vi "Build Sparse Array.vi"(4 "Side":T1=enum."right") -> ()   [LabVIEW 2013]
uses:
  ROS/Code/SubVIs/BaxterSide.ctl
  Baxter Examples/Arm Globals.vi
  <vilib>/Utility/config.llb/Read Key (Double).vi
  Fwd Kenimatics - array.vi
  <vilib>/Utility/config.llb/NI_LVConfig.lvlib
panel:
  out "output variable":dbl
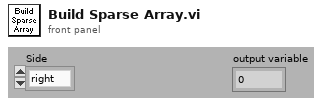
[diagram p1: front panel]
types:
  T1 = typedef "BaxterSide.ctl" = enum16{"left", "right"}
  T2 = cluster{"J[0]":dbl, "J[1]":dbl, "J[2]":dbl, "J[3]":dbl, "J[4]":dbl, "J[5]":dbl, "J[6]":dbl}
  T3 = cluster{"Label":string, "Joints":dbl[], "Far Left":cluster{"Absolute":dbl[], "Robot":dbl[]}, "Far Right":cluster{"Absolute":dbl[], "Robot":dbl[]}, "Near Left":cluster{"Absolute":dbl[], "Robot":dbl[]}, "Near Right":cluster{"Absolute":dbl[], "Robot":dbl[]}}[]
  T4 = typedef "NI_Matrix.lvlib/RealMatrix.ctl" = dbl[][]
  T5 = cluster{"Label":string, "Joints":dbl[], "T":T4}[]
  T6 = typedef "NI_LVConfig.lvlib/Config Data RefNum.ctl" = refnum<k1>
  T7 = cluster{"J[0]":dbl, "J[1]":dbl, "J[2]":dbl, "J[3]":dbl, "J[4]":dbl, "J[5]":dbl, "J[6]":dbl}[]
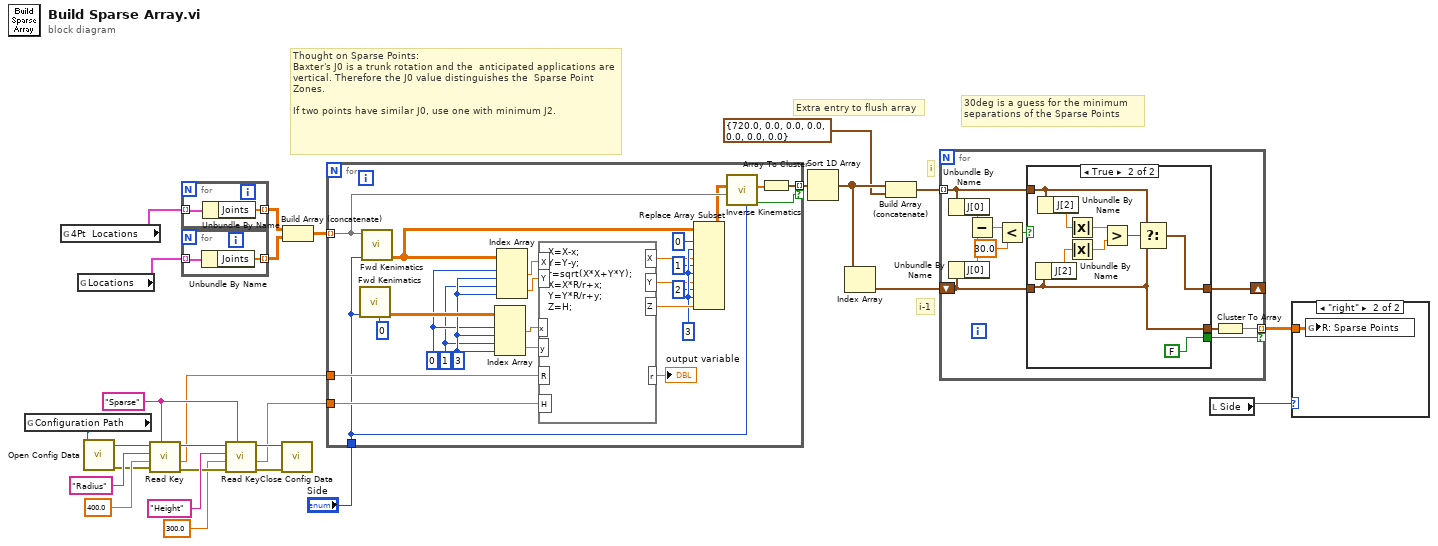
[diagram p0: block diagram]
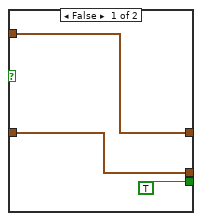
[diagram p3: hidden frame]
diagram:
  w23 = "Sparse"
  # "30deg is a guess for the minimum\nseparations of the Sparse Points"
  # "Extra entry to flush array"
  # "i-1"
  # "i"
  # "Thought on Sparse Points:\nBaxter's J0 is a trunk rotation and the  anticipated applications are vertical. Therefore the J0 value distinguishes the  Sparse Point Zones.\n\nIf two points have similar J0, use one with minimum J2."
  n1 = global read "Arm Globals.vi" "Configuration Path"() -> (w27:path)
  n2 = global read "Arm Globals.vi" "4Pt  Locations"() -> (w13:T3)
  n3 = global read "Arm Globals.vi" "Locations"() -> (w12:T5)
  n4 = call <vilib>:"Open Config Data.vi"("configuration file path"=w27) -> ("error out"=w20:errorcluster, "refnum"=w26:T6)  [unwired: 8 in, 1 out]
  n5 = call-poly <vilib>:"Read Key.vi"("section"=w23, "error in (no error)"=w20, "default value"=400.0, "key"="Radius", "refnum"=w26) -> ("error out"=w19:errorcluster, "value"=w15:dbl, "refnum out"=w24:T6)  [unwired: 3 in, 1 out]
  n6 = for {
    tunnel: w13 -> [w29] mode=indexing
    tunnel: [w28] -> w11 mode=indexing
    n7 = Unbundle By Name(w29) -> ("Joints"=w28:dbl[])
  }
  n8 = for {
    tunnel: w12 -> [w31] mode=indexing
    tunnel: [w30] -> w10 mode=indexing
    n9 = Unbundle By Name(w31) -> ("Joints"=w30:dbl[])
  }
  n10 = call-poly <vilib>:"Read Key.vi"("section"=w23, "error in (no error)"=w19, "default value"=300.0, "key"="Height", "refnum"=w24) -> ("error out"=w16:errorcluster, "value"=w14:dbl, "refnum out"=w17:T6)  [unwired: 3 in, 1 out]
  n11 = call <vilib>:"Close Config Data.vi"("error in (no error)"=w16, "refnum"=w17) -> ()  [unwired: 8 in, 2 out]
  n12 = Build Array (concatenate)(w11, w10) -> (w9:dbl[][])
  n13 = for {
    tunnel: w15 -> [w54]
    tunnel: w14 -> [w51]
    tunnel: w9 -> [w45] mode=indexing
    tunnel: "Side" -> [w33]
    tunnel: [w41] -> w8 mode=indexing if=w40
    w35 = 1 ("disabled index (row)")
    w36 = 0 ("disabled index (row)")
    w37 = 3 ("disabled index (col)")
    w48 = 3 ("disabled index (col)")
    n14 = call-poly "Fwd Kenimatics.vi"("To"=0, "Side"=w33) -> ("Matrix"=w38:T4)  [unwired: 8 in, 1 out]
    n15 = call-poly "Fwd Kenimatics.vi"("Side"=w33, "Joints"=w45) -> ("Matrix"=w34:T4)  [unwired: 8 in, 1 out]
    n16 = Index Array(array=w38, index (row) #1=w36, index (col) #1=w37, index (row) #2=w35, index (col) #2=w37) -> (element #1=w52:dbl, element #2=w53:dbl)
    n17 = Index Array(array=w34, index (row) #1=w36, index (col) #1=w37, index (row) #2=w35, index (col) #2=w37) -> (element #1=w56:dbl, element #2=w55:dbl)
    n18 = formula code="X=X-x;\nY=Y-y;\nr=sqrt(X*X+Y*Y);\nX=X*R/r+x;\nY=Y*R/r+y;\nZ=H;"("R"=w54, "X"=w56, "Y"=w55, "x"=w52, "y"=w53, "H"=w51) -> ("r"=→"output variable":dbl, "X"=w44:dbl, "Y"=w43:dbl, "Z"=w50:dbl)
    n19 = Replace Array Subset(array=w34, new element #1=w44, index (row) #1=0 ("disabled index (row)"), index (col) #1=w48, new element #2=w43, index (row) #2=1 ("disabled index (row)"), index (col) #2=w48, new element #3=w50, index (row) #3=2 ("disabled index (row)"), index (col) #3=w48) -> (w32:T4)
    n20 = call "Inverse Kinematics.vi"("Side"=w33, "Start"=w45, "Goal-matrix"=w32) -> ("Found"=w40:bool, "J"=w42:dbl[])  [unwired: 5 in, 2 out]
    n21 = Array To Cluster(array=w42) -> (cluster=w41:T2)
  }
  n22 = Sort 1D Array(array=w8) -> (sorted array=w6:T7)
  n23 = Index Array(array=w6) -> (element=w7:T2)  [unwired: 1 in]
  n24 = Build Array (concatenate)(w6, T2 {"J[0]"=720.0, "J[1]"=0.0, "J[2]"=0.0, "J[3]"=0.0, "J[4]"=0.0, "J[5]"=0.0, "J[6]"=0.0} ("cluster")) -> (w4:T7)
  n25 = for {
    tunnel: w4 -> [w62] mode=indexing
    tunnel: [w68] -> w1 mode=indexing if=w59
    shift-right: [w58] -> _
    shift-left: w7 -> [w61]
    n26 = Unbundle By Name(w62) -> ("J[0]"=w65:dbl)
    n27 = Unbundle By Name(w61) -> ("J[0]"=w64:dbl)
    n28 = Subtract(x=w65, y=w64) -> (x-y=w67:dbl)
    n29 = Less?(x=w67, y=30.0) -> (x < y?=w63:bool)
    n30 = case shown="True" w63 {
      tunnel: w62 -> [w69 w74]
      tunnel: w61 -> [w71 w73]
      tunnel: [w71 w73] -> w60
      tunnel: [TRUE FALSE] -> w59
      tunnel: [w69 w72] -> w58
      frame False {
      }
      frame True {
        n31 = Unbundle By Name(w73) -> ("J[2]"=w78:dbl)
        n32 = Unbundle By Name(w74) -> ("J[2]"=w79:dbl)
        n33 = Absolute Value(x=w79) -> (abs(x)=w77:dbl)
        n34 = Absolute Value(x=w78) -> (abs(x)=w76:dbl)
        n35 = Greater?(x=w77, y=w76) -> (0:w75:bool)
        n36 = Select(t=w74, s=w75, f=w73) -> (s? t:f=w72:T2)
      }
    }
    n37 = Cluster To Array(cluster=w60) -> (array=w68:dbl[])
  }
  n38 = local read "Side"() -> (w2:T1)
  n39 = case shown="\"right\"" w2 {
    tunnel: w1 -> [_ w81]
    frame "left", Default {
    }
    frame "right" {
      n40 = global write "Arm Globals.vi" "R: Sparse Points"(w81) -> ()
    }
  }
